vi "Fit VI window to Visible Content.vi"(4 "error in (no error)":errorcluster, 6 "border spacing (2 px)":i32=2, 7 "VI Ref":refnum<vi>) -> (0 "error out":errorcluster, 3 "dup VI Ref":refnum<vi>)   [LabVIEW 2017, in "csm-ui-support.lvlib"]
doc: "This utility will fit (resize and center) a VI (defined by the \"VI Ref\" input) about the all of the Front Panel object. It will add a border defined by border spacing in units of pixels. If no VI Reference is passed in, it will operate on the calling VI."
uses:
  csm-ui-support.lvlib
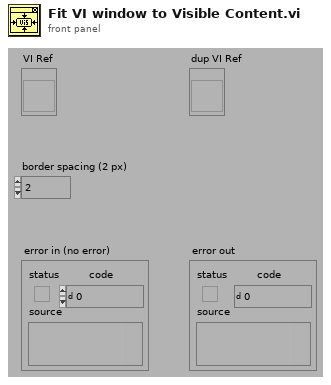
[diagram p1: front panel]
types:
  T1 = typedef "LVRectTypeDef.ctl" = cluster{"Left":i16, "Top":i16, "Right":i16, "Bottom":i16}
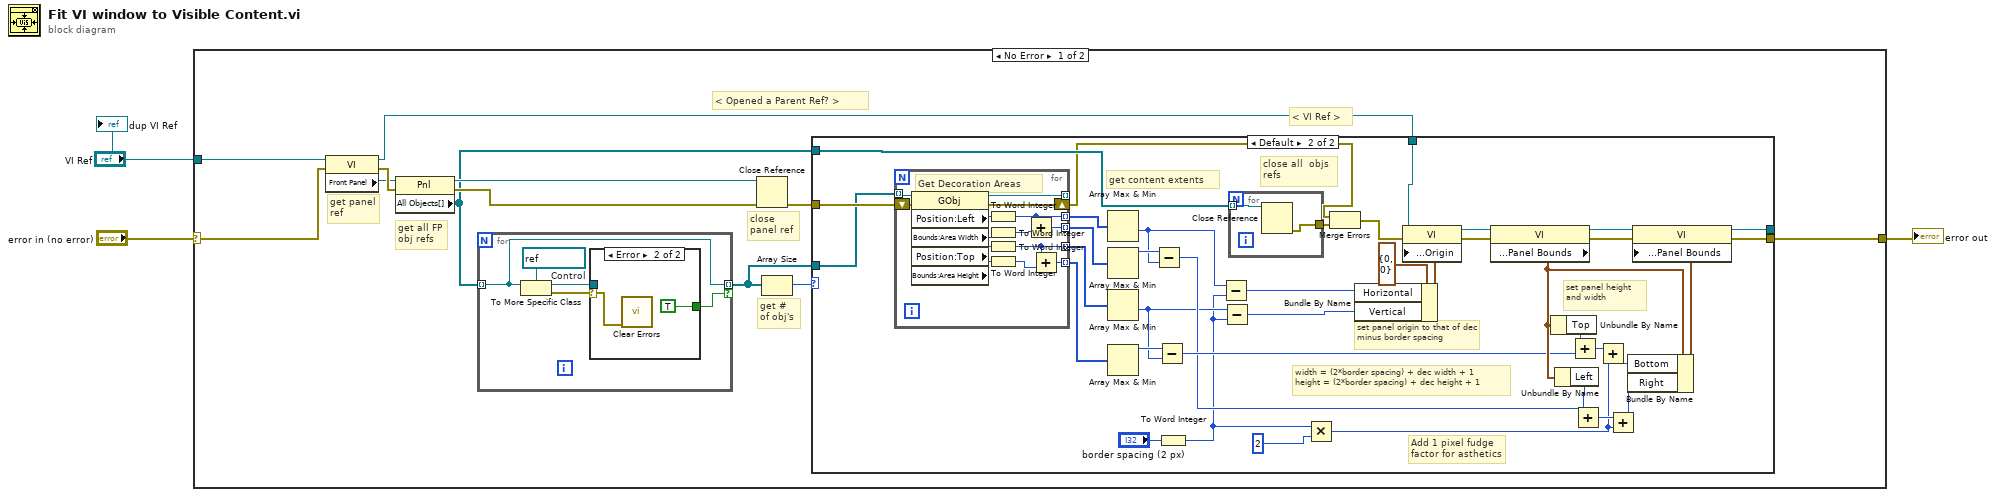
[diagram p0: block diagram]
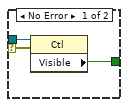
[diagram p2: hidden frame]
diagram:
  n1 = case shown="No Error" "error in (no error)" {
    selector: "error in (no error)" -> [w7 w83]
    tunnel: [w9 w83] -> w3
    tunnel: "VI Ref" -> [w4 _]
    frame No Error {
      # "< Opened a Parent Ref? >"
      # "get # of obj's"
      # "get panel ref"
      # "get all FP obj refs"
      # "close panel ref"
      # "< VI Ref >"
      n2 = property on="Property Node" class="VI"(reference=w4, error in=w7) -> (reference out=w15:refnum<vi>, error out=w13:errorcluster, "Front Panel"=w11:refnum<vi>)
      n3 = property on="Property Node" class="Pnl"(reference=w11, error in=w13) -> (reference out=w14:refnum<vi>, error out=w12:errorcluster, "All Objects[]"=w6:refnum<vi>[])
      n4 = for {
        tunnel: [w16] -> w5 mode=indexing if=w17
        tunnel: w6 -> [w16] mode=indexing
        w19 = refnum<vi> refnum  # Control
        n5 = To More Specific Class(target class=w19, reference=w16) -> (specific class reference=w20:refnum<vi>, error out=w18:errorcluster)  [unwired: 1 in]
        n6 = case shown="Error" w18 {
          selector: w18 -> [w22 w24]
          tunnel: w20 -> [w23 _]
          tunnel: [w21 TRUE ("Visible")] -> w17
          frame No Error {
            n7 = property class="Ctl"(reference=w23, error in=w22) -> ("Visible"=w21:bool)  [unwired: 2 out]
          }
          frame Error {
            n8 = call <vilib>:"Clear Errors.vi"("error in (no error)"=w24) -> ()  [unwired: 5 in, 2 out]
          }
        }
      }
      n9 = Close Reference(reference=w14, error in (no error)=w12) -> (error out=w10:errorcluster)
      n10 = Array Size(array=w5) -> (size(s)=w8:i32)
      n11 = case shown="Default" w8 {
        tunnel: w15 -> [w27 w64]
        tunnel: w10 -> [w26 w51]
        tunnel: [w26 w46] -> w9
        tunnel: [w27 w45] -> _
        tunnel: w6 -> [_ w31]
        tunnel: w5 -> [_ w30]
        frame 0 {
          # "do nothing if no objects"
        }
        frame Default {
          # "width = (2*border spacing) + dec width + 1\nheight = (2*border spacing) + dec height + 1"
          # "set panel height and width"
          # "set panel origin to that of dec minus border spacing"
          # "close all  objs refs"
          # "get content extents"
          # "Add 1 pixel fudge factor for asthetics"
          n12 = for {
            tunnel: w30 -> [w82] mode=indexing
            shift-right: [w80] -> w28
            shift-left: w51 -> [w81]
            tunnel: [w79] -> _ mode=indexing
            tunnel: [w75] -> w43 mode=indexing
            tunnel: [w77] -> w42 mode=indexing
            tunnel: [w71] -> w41 mode=indexing
            tunnel: [w76] -> w40 mode=indexing
            # "Get Decoration Areas"
            n13 = property class="GObj"(reference=w82, error in=w81) -> (reference out=w79:refnum<vi>, error out=w80:errorcluster, "Position:Left"=w78:i32, "Bounds:Area Width"=w74:u32, "Position:Top"=w72:i32, "Bounds:Area Height"=w70:u32)
            n14 = To Word Integer(number=w78) -> (16bit integer=w75:i16)
            n15 = To Word Integer(number=w74) -> (16bit integer=w73:i16)
            n16 = To Word Integer(number=w72) -> (16bit integer=w71:i16)
            n17 = To Word Integer(number=w70) -> (16bit integer=w69:i16)
            n18 = Add(x=w75, y=w73) -> (x+y=w77:i16)
            n19 = Add(x=w71, y=w69) -> (x+y=w76:i16)
          }
          n20 = Array Max & Min(array=w43) -> (min value=w34:i16)  [unwired: 3 out]
          n21 = Array Max & Min(array=w42) -> (max value=w37:i16)  [unwired: 3 out]
          n22 = Array Max & Min(array=w41) -> (min value=w35:i16)  [unwired: 3 out]
          n23 = Array Max & Min(array=w40) -> (max value=w39:i16)  [unwired: 3 out]
          n24 = Subtract(x=w37, y=w34) -> (x-y=w36:i16)
          n25 = Subtract(x=w39, y=w35) -> (x-y=w38:i16)
          n26 = To Word Integer(number="border spacing (2 px)") -> (16bit integer=w32:i16)
          n27 = Subtract(x=w34, y=w32) -> (x-y=w54:i16)
          n28 = Subtract(x=w35, y=w32) -> (x-y=w55:i16)
          n29 = for {
            tunnel: w31 -> [w67] mode=indexing
            tunnel: [w68] -> w33
            n30 = Close Reference(reference=w67) -> (error out=w68:errorcluster)  [unwired: 1 in]
          }
          n31 = Multiply(x=w32, y=i16 2) -> (x*y=w44:i16)
          n32 = Merge Errors(w28, w33) -> (w29:errorcluster)
          n33 = Bundle By Name(cluster=cluster{"Horizontal":i16, "Vertical":i16} {"Horizontal"=0, "Vertical"=0} ("Front Panel Window:Origin"), "Horizontal"=w54, "Vertical"=w55) -> (w52:cluster{"Horizontal":i16, "Vertical":i16})
          n34 = property on="Property Node" class="VI"(reference=w64, error in=w29, "Front Panel Window:Origin"=w52) -> (reference out=w65:refnum<vi>, error out=w48:errorcluster)
          n35 = property on="Property Node" class="VI"(reference=w65, error in=w48) -> (reference out=w66:refnum<vi>, error out=w47:errorcluster, "Front Panel Window:Panel Bounds"=w56:T1)
          n36 = Unbundle By Name(w56) -> ("Top"=w57:i16)
          n37 = Unbundle By Name(w56) -> ("Left"=w58:i16)
          n38 = Add(x=w57, y=w38) -> (x+y=w62:i16)
          n39 = Add(x=w58, y=w36) -> (x+y=w60:i16)
          n40 = Add(x=w62, y=w44) -> (x+y=w63:i16)
          n41 = Add(x=w60, y=w44) -> (x+y=w61:i16)
          n42 = Bundle By Name(cluster=w56, "Bottom"=w63, "Right"=w61) -> (w59:T1)
          n43 = property on="Property Node" class="VI"(reference=w66, error in=w47, "Front Panel Window:Panel Bounds"=w59) -> (reference out=w45:refnum<vi>, error out=w46:errorcluster)
        }
      }
    }
    frame Error {
    }
  }
  "error out" <- w3
  "dup VI Ref" <- "VI Ref"
